vi "OSSCAR_v3_BM.vi"() -> ()   [LabVIEW 2021]
uses:
  SubVIs/Global_stop.vi
  SubVIs/Plot_trap_heating_global_BM.vi
  SubVIs/OSSCAR_stop_global_BM.vi
  SubVIs/DMSO-related/Temp_global_BM.vi
panel:
  in  "N Interval Pt. Std.s":dbl=6.0 caption="Every"
  in  "Interval Pt. Std.?":bool
  in  "Runtype":enum16{"Single", "Continuous"}(ring)
  in  "Program Control":bool caption="Program Stop"
  out "Current Std #":string
  out "Current Analyte:":string="DMS"
  in  "N std pt.s":i32=6
  in  "Mode Selection":T1(ring)
  in  "Standalone Function":T2(ring)=enum."Condition Trap"
  out "Reduction Countdown (min)":dbl format="%.2g"
  out "Hydrolysis Countdown (min)":dbl format="%.2g"
  out "Sparge Countdown (min)":dbl format="%.2g"
  out "Elution Countdown (min)":dbl format="%.2f"
  out "Hydrolysis Progress Bar":u8(slide)=100 scale=0.0..100.0
  out "Reduction Progress Bar":u8(slide)=100 scale=0.0..100.0
  out "Elution Progress Bar":u8(slide)=100 scale=0.0..100.0
  out "Sparging Progress Bar":u8(slide)=100 scale=0.0..100.0
  in  "Analysis Type":T3(ring)
  in  "Tab Control":T4(tab)
  in  "Metadata":T5={"Local save location:"="C:\\Users\\LabPC1\\OneDrive\\Desktop\\OSSCAR_metadata\\Test_metadata", "Cruise ID"="LaPerouse", "Sampling Timestamp"="2023-07-19 15:23:13", "Elution Timestamp"="2023-07-19 15:29:12", "GPS_Latitude"=-999.0, "GPS_Longitude"=-999.0, "DMS_std_conc"=0.0, "DMSP_std_conc"=0.0, "DMSO_std_conc"=0.0, "Std_index"=0.0, "Initial Trap Temp (oC)"=29.0, "Max Trap Temp (oC)"=161.0, "Final Trap Temp (oC)"=31.0, "Flow Rate (mL/min)"=0.0, "Comment"="", "GPS_Minute"=-999.0, "GPS_Day"=-999.0, "GPS_jd"=-999.0, "GPS_Hour"=-999.0, "GPS_Second"=-999.0, "GPS Baud"=4800.0, "COM Port (GPS)"="COM10", "Use GPS?"=FALSE, "Format Date"="%d-%d-%d"} {"GPS_Latitude" format="%_4g"; "GPS_Longitude" format="%_4g"; "GPS_jd" format="%_5g"; "Std_index" format="%.2g"; "DMSO_std_conc" format="%.2f"; "DMSP_std_conc" format="%.2f"; "DMS_std_conc" format="%.2f"}
  in  "Sample Params":T6={"DMS Sparge Time (min)"=7.0, "Elution Time (min)"=1.5, "COM port (16 Pos. Valve)"="COM10", "Trap Heating Time (ms)"=900.0, "COM Port (DC Power)"="COM5", "COM Port (Runze)"="COM4", "Sample Vol (mL)"=10.0, "DMSO Red. Duration (min)"=30.0, "Bypass sample handling (debugging)"=FALSE, "Reverse Reduction?"=FALSE, "Voltage (V)"="4.0", "DMSP Hydrolysis Time (min)"=13.0, "Total Vol. (mL)"=10.0, "Split DMSP sample?"=TRUE, "Remove DMSP vol. (mL)"=5.0}
  in  "Constants":T7={"step to ml"=1920.0, "BoardNum"=0, "PosA BitNum"=1, "PosB BitNum"=2, "Heat Pulse Delay (ms)"=0.0, "Heating Iterations"=12, "N rinses"=2, "Dissolution Time (s)"=120, "SpargeBit"=0, "Extra Milli-Q (ml)"=2.0, "Valco Port Number"=6, "BitNum (Thermocouple)"=1, "N syringe rinses"=2, "NaOH Vol (ml)"=2.0, "FanBit"=4}
  in  "Pump Parameters":T8={"Speed 1"="100", "Speed 2"="250", "Speed 3"="350", "Speed 4"="250", "UW/Sample"="5", "Sparge"="2", "Std"="4", "Waste"="15", "Air"="14", "Milli-Q"="1", "H2SO4"="6", "NaOH"="3", "Catalyst"="7", "Cell (H+ side)"="8", "Cell (sample side)"="9", "NaCl"="11"}
  out "Current Temp:":i32=31
  out "Trap Heating":cluster{"Y":dbl[], "Y":dbl[]}[](graph)
  # "OSSCAR DMS/O/P Program"
  # "Runs"
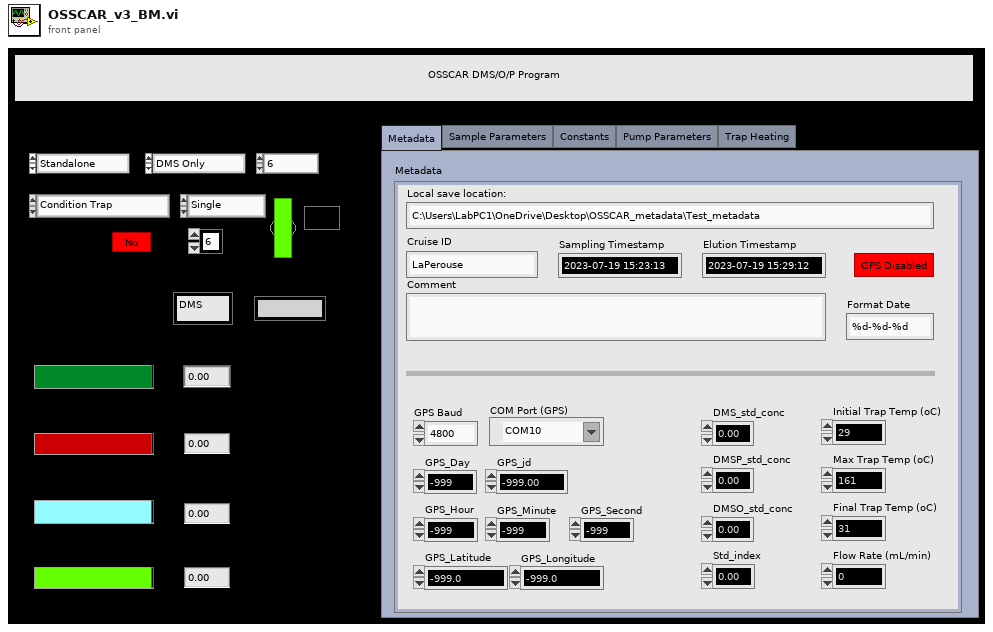
[diagram p1: front panel]
types:
  T1 = enum16{"Standalone", "Analysis", "Standard Curve", "Point Std"}
  T2 = enum16{"Send Pump Command", "Condition Trap", "Control Fan", "Control Sparger", "Load/Inject Trap", "Switch Flow Path", "Control cell DC power", "Rinse Sparge Chamber", "Rinse Cell"}
  T3 = enum16{"DMS Only", "DMS/O", "DMS/P", "DMS/O/P", "DMSO Only"}
  T4 = enum32{"Metadata", "Sample Parameters", "Constants", "Pump Parameters", "Trap Heating"}
  T5 = cluster{"Local save location:":string, "Cruise ID":string, "Sampling Timestamp":string, "Elution Timestamp":string, "GPS_Latitude":dbl, "GPS_Longitude":dbl, "DMS_std_conc":dbl, "DMSP_std_conc":dbl, "DMSO_std_conc":dbl, "Std_index":dbl, "Initial Trap Temp (oC)":dbl, "Max Trap Temp (oC)":dbl, "Final Trap Temp (oC)":dbl, "Flow Rate (mL/min)":dbl, "Comment":string, "GPS_Minute":dbl, "GPS_Day":dbl, "GPS_jd":dbl, "GPS_Hour":dbl, "GPS_Second":dbl, "GPS Baud":dbl, "COM Port (GPS)":refnum<visa-resource-name>, "Use GPS?":bool, "Format Date":string}
  T6 = cluster{"DMS Sparge Time (min)":dbl, "Elution Time (min)":dbl, "COM port (16 Pos. Valve)":refnum<visa-resource-name>, "Trap Heating Time (ms)":dbl, "COM Port (DC Power)":refnum<visa-resource-name>, "COM Port (Runze)":refnum<visa-resource-name>, "Sample Vol (mL)":dbl, "DMSO Red. Duration (min)":dbl, "Bypass sample handling (debugging)":bool, "Reverse Reduction?":bool, "Voltage (V)":string, "DMSP Hydrolysis Time (min)":dbl, "Total Vol. (mL)":dbl, "Split DMSP sample?":bool, "Remove DMSP vol. (mL)":dbl}
  T7 = cluster{"step to ml":dbl, "BoardNum":u32, "PosA BitNum":u32, "PosB BitNum":u32, "Heat Pulse Delay (ms)":dbl, "Heating Iterations":i32, "N rinses":i32, "Dissolution Time (s)":u32, "SpargeBit":u32, "Extra Milli-Q (ml)":dbl, "Valco Port Number":i32, "BitNum (Thermocouple)":u32, "N syringe rinses":i32, "NaOH Vol (ml)":dbl, "FanBit":u32}
  T8 = cluster{"Speed 1":string, "Speed 2":string, "Speed 3":string, "Speed 4":string, "UW/Sample":string, "Sparge":string, "Std":string, "Waste":string, "Air":string, "Milli-Q":string, "H2SO4":string, "NaOH":string, "Catalyst":string, "Cell (H+ side)":string, "Cell (sample side)":string, "NaCl":string}
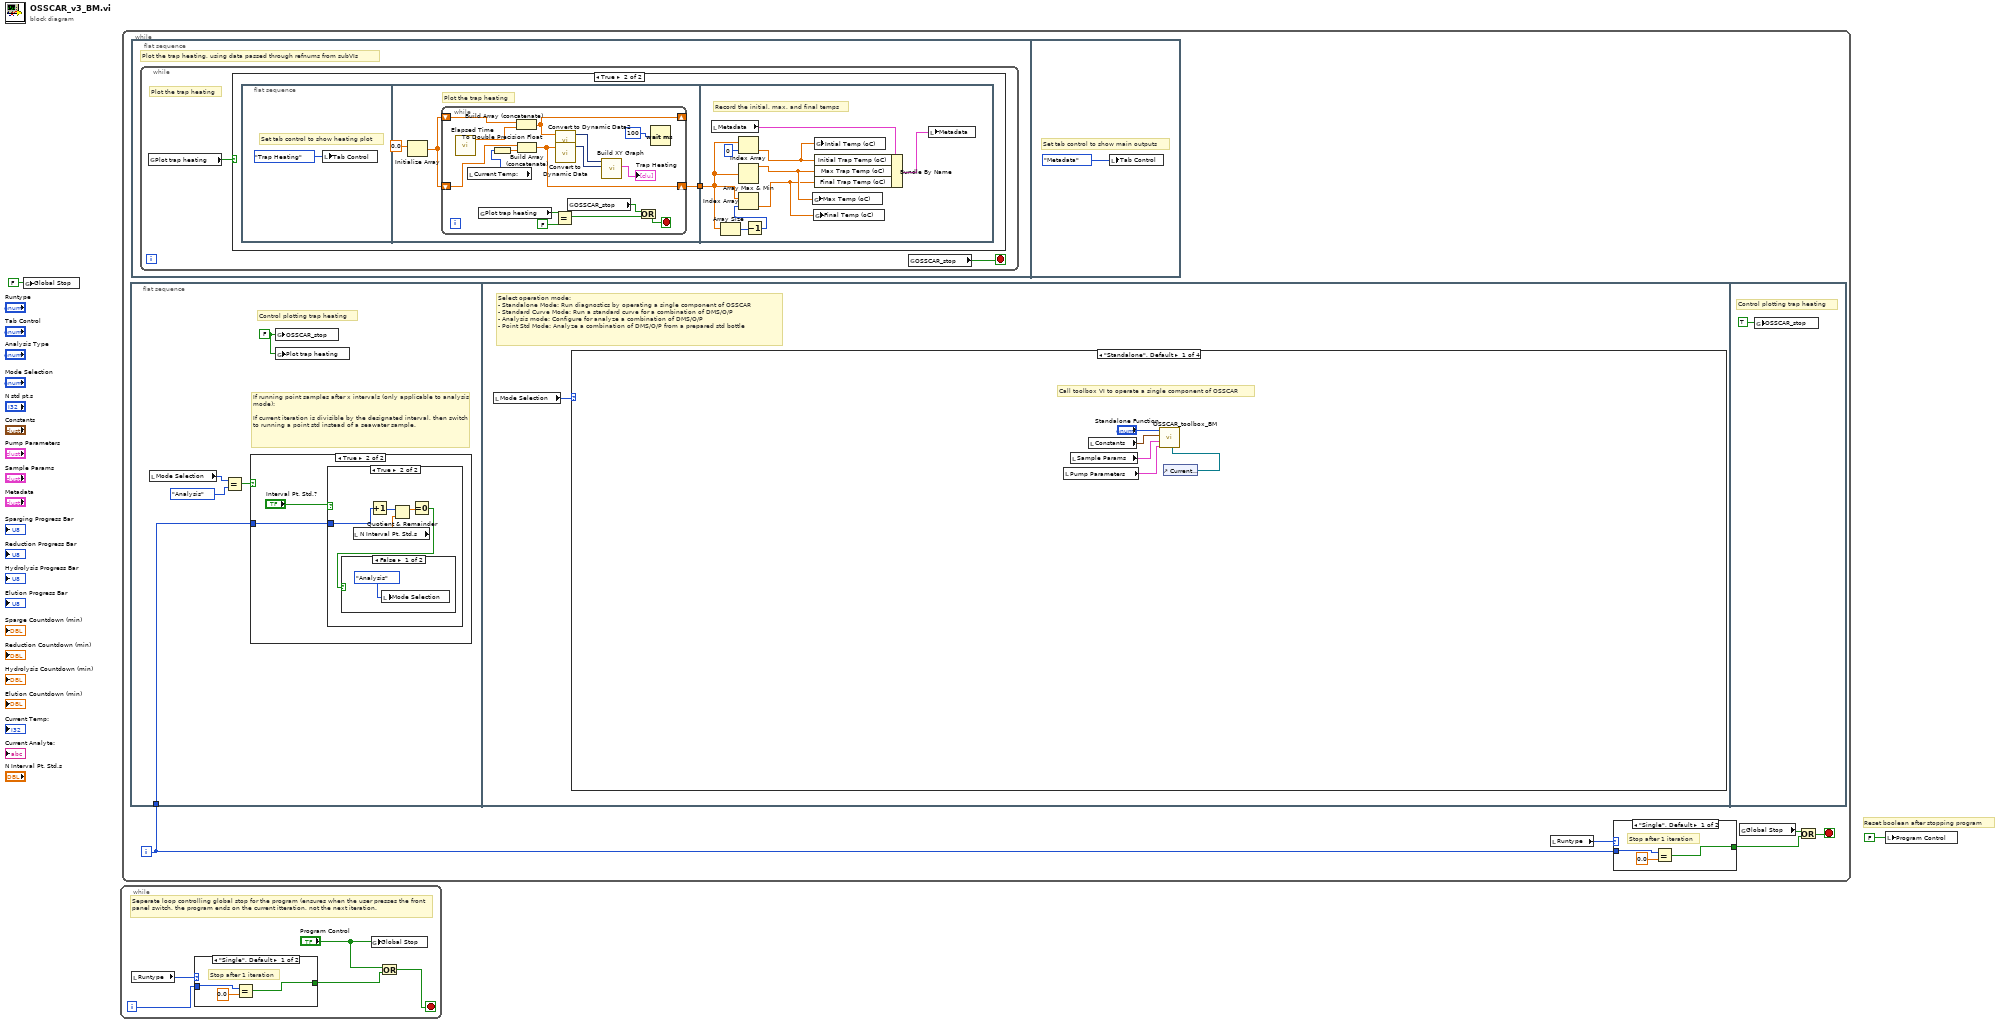
[diagram p0: block diagram]
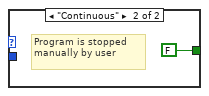
[diagram p2: hidden frame]
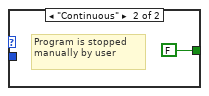
[diagram p4: hidden frame]
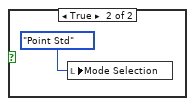
[diagram p7: hidden frame]
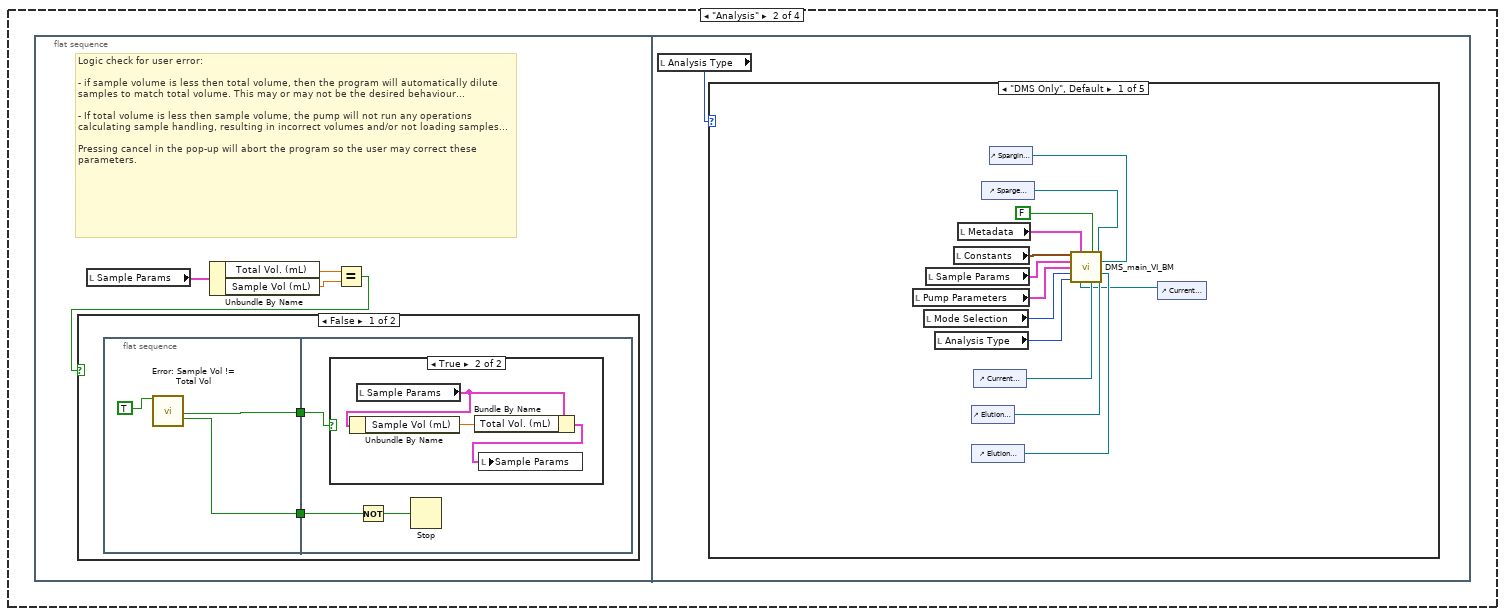
[diagram p8: hidden frame]
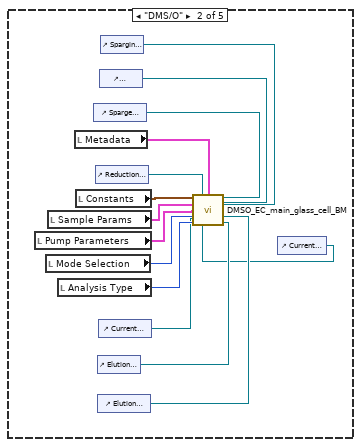
[diagram p11: hidden frame]
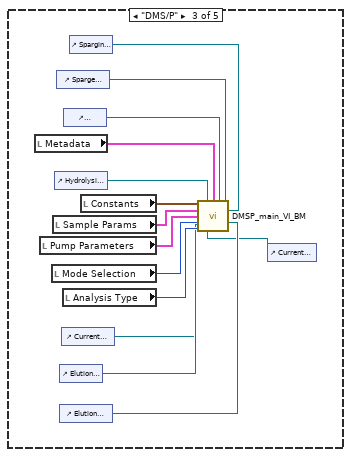
[diagram p12: hidden frame]
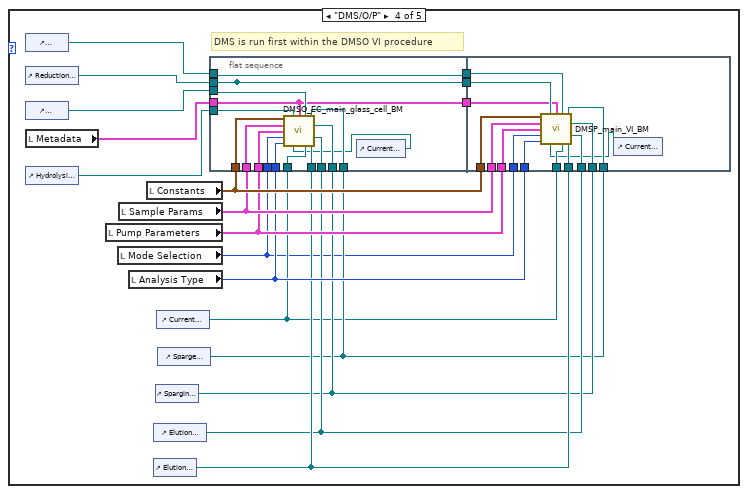
[diagram p13: hidden frame]
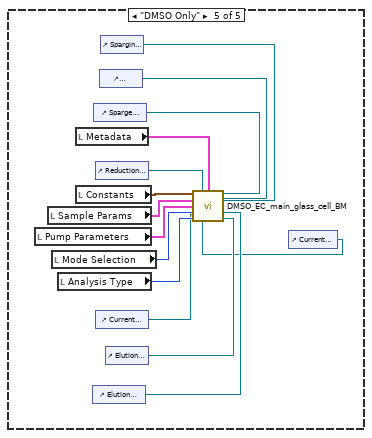
[diagram p14: hidden frame]
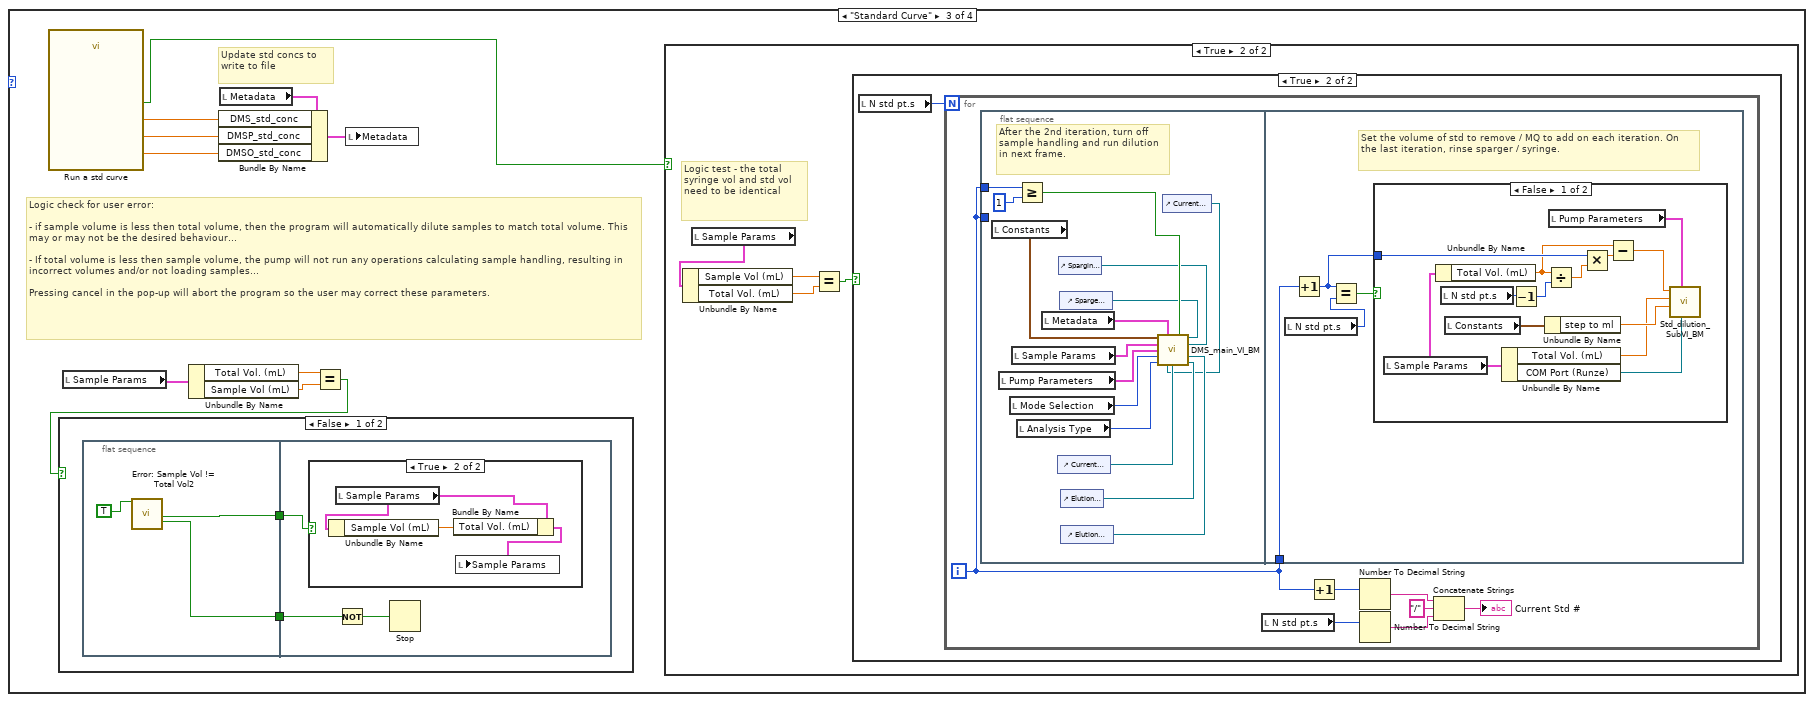
[diagram p15: hidden frame]
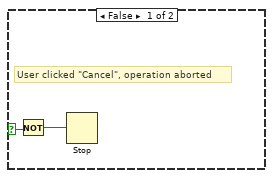
[diagram p18: hidden frame]
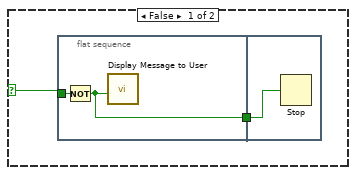
[diagram p19: hidden frame]
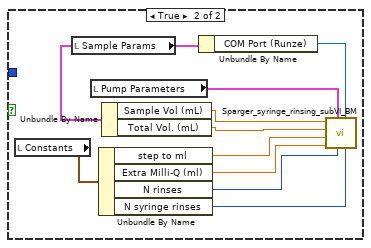
[diagram p20: hidden frame]
diagram:
  # "Reset boolean after stopping program"
  n1 = global write "Global_stop.vi" "Global Stop"(FALSE ("Global Stop")) -> ()
  n2 = while {
    i -> [w3]
    stop <- w4 stop-if-true
    # "Seperate loop controlling global stop for the program (ensures when the user presses the front panel switch, the program ends on the current itteration, not the next iteration."
    n3 = local read "Runtype"() -> (w7:enum16{"Single", "Continuous"})
    n4 = case shown="\"Single\", Default" w7 {
      tunnel: w3 -> [w9 _]
      tunnel: [w8 FALSE] -> w6
      frame "Single", Default {
        # "Stop after 1 iteration"
        n5 = Equal?(x=w9, y=0.0) -> (x = y?=w8:bool)
      }
      frame "Continuous" {
        # "Program is stopped manually by user"
      }
    }
    n6 = global write "Global_stop.vi" "Global Stop"("Program Control") -> ()
    n7 = Or(x="Program Control", y=w6) -> (x .or. y?=w4:bool)
  }
  n8 = while {
    i -> [w15]
    stop <- w14 stop-if-true
    n9 = flat-sequence {
      tunnel: w15 -> [w57]
      frame #0 {
        w58 = FALSE ("OSSCAR_stop")
        # "If running point samples after x intervals (only applicable to analysis mode):\n\nIf current iteration is divisible by the designated interval, then switch to running a point std instead of a seawater sample."
        # "Control plotting trap heating"
        n10 = local read "Mode Selection"() -> (w55:T1)
        n11 = Equal?(x=w55, y=T1."Analysis" ("Mode Selection")) -> (x = y?=w56:bool)
        n12 = case shown="True" w56 {
          tunnel: w57 -> [_ w60]
          frame False {
            # "Not running analysis / point std, proceed with other operations"
          }
          frame True {
            n13 = case shown="True" "Interval Pt. Std.?" {
              tunnel: w60 -> [_ w61]
              frame False {
                # "Not running point stds, so continue with analysis"
              }
              frame True {
                n14 = local read "N Interval Pt. Std.s"() -> (w65:dbl)
                n15 = Increment(x=w61) -> (x+1=w62:i32)
                n16 = Quotient & Remainder(x=w62, y=w65) -> (x-y*floor(x/y)=w64:dbl)  [unwired: 1 out]
                n17 = Equal To 0?(x=w64) -> (x = 0?=w63:bool)
                n18 = case shown="False" w63 {
                  frame False {
                    n19 = local write "Mode Selection"(T1."Analysis" ("Mode Selection")) -> ()
                  }
                  frame True {
                    n20 = local write "Mode Selection"(T1."Point Std" ("Mode Selection")) -> ()
                  }
                }
              }
            }
          }
        }
        n21 = global write "OSSCAR_stop_global_BM.vi" "OSSCAR_stop"(w58) -> ()
        n22 = global write "Plot_trap_heating_global_BM.vi" "Plot trap heating"(w58) -> ()
      }
      frame #1 {
        # "Select operation mode:\n- Standalone Mode: Run diagnostics by operating a single component of OSSCAR\n- Standard Curve Mode: Run a standard curve for a combination of DMS/O/P\n- Analysis mode: Configure for analyze a combination of DMS/O/P\n- Point Std Mode: Analyze a combination of DMS/O/P from a prepared std bottle"
        n23 = local read "Mode Selection"() -> (w68:T1)
        n24 = case shown="\"Standalone\", Default" w68 {
          frame "Standalone", Default {
            # "Call toolbox VI to operate a single component of OSSCAR"
            n25 = local read "Pump Parameters"() -> (w69:T8)
            n26 = local read "Sample Params"() -> (w70:T6)
            n27 = local read "Constants"() -> (w71:T7)
            n28 = control-ref of="Current Temp:"() -> (w72:refnum<vi>)
            n29 = call "OSSCAR_toolbox_BM.vi"("Temp Refnum"=w72, "Pump Parameters"=w69, "Sample Params"=w70, "Constants"=w71, "Function"="Standalone Function") -> ()  [unwired: 7 in]
          }
          frame "Analysis" {
            n30 = flat-sequence {
              frame #0 {
                # "Logic check for user error:\n\n- if sample volume is less then total volume, then the program will automatically dilute samples to match total volume. This may or may not be the desired behaviour...\n\n- If total volume is less then sample volume, the pump will not run any operations calculating sample handling, resulting in incorrect volumes and/or not loading samples...\n\nPressing cancel in the pop-up will abort the program so the user may correct these parameters."
                n31 = local read "Sample Params"() -> (w77:T6)
                n32 = Unbundle By Name(w77) -> ("Total Vol. (mL)"=w74:dbl, "Sample Vol (mL)"=w76:dbl)
                n33 = Equal?(x=w74, y=w76) -> (x = y?=w75:bool)
                n34 = case shown="False" w75 {
                  frame False {
                    n35 = flat-sequence {
                      tunnel: [w82] -> w79
                      tunnel: [w81] -> w78
                      tunnel: w79 -> [w85]
                      tunnel: w78 -> [w83]
                      frame #0 {
                        n36 = call "Error: Sample Vol != Total Vol"("Enable"=TRUE) -> ("Make Total Vol = Sample Vol?"=w81:bool, "Proceed"=w82:bool)  [unwired: 16 in, 1 out]
                      }
                      frame #1 {
                        n37 = case shown="True" w83 {
                          frame False {
                            # "User indicated sample vol should not equal total vol, continue to analysis."
                          }
                          frame True {
                            n38 = local read "Sample Params"() -> (w87:T6)
                            n39 = Unbundle By Name(w87) -> ("Sample Vol (mL)"=w88:dbl)
                            n40 = Bundle By Name(cluster=w87, "Total Vol. (mL)"=w88) -> (w86:T6)
                            n41 = local write "Sample Params"(w86) -> ()
                          }
                        }
                        n42 = Not(x=w85) -> (.not. x?=w84:bool)
                        n43 = Stop(stop? (T)=w84) -> ()
                      }
                    }
                  }
                  frame True {
                    # "Else: carry on, nothing to see here..."
                  }
                }
              }
              frame #1 {
                n44 = local read "Analysis Type"() -> (w89:T3)
                n45 = case shown="\"DMS Only\", Default" w89 {
                  frame "DMS Only", Default {
                    n46 = local read "Pump Parameters"() -> (w101:T8)
                    n47 = local read "Mode Selection"() -> (w90:T1)
                    n48 = local read "Sample Params"() -> (w102:T6)
                    n49 = local read "Analysis Type"() -> (w100:T3)
                    n50 = local read "Constants"() -> (w93:T7)
                    n51 = local read "Metadata"() -> (w92:T5)
                    n52 = control-ref of="Elution Progress Bar"() -> (w95:refnum<vi>)
                    n53 = control-ref of="Elution Countdown (min)"() -> (w96:refnum<vi>)
                    n54 = control-ref of="Current Temp:"() -> (w94:refnum<vi>)
                    n55 = control-ref of="Sparge Countdown (min)"() -> (w98:refnum<vi>)
                    n56 = control-ref of="Sparging Progress Bar"() -> (w97:refnum<vi>)
                    n57 = control-ref of="Current Analyte:"() -> (w91:refnum<vi>)
                    n58 = call "DMS_main_VI_BM.vi"("Constants"=w93, "Metadata"=w92, "Skip sample handling"=FALSE, "Sparging Countdown Timer Refnum"=w98, "Sample Params"=w102, "Sparging Progress Bar Refnum"=w97, "Pump Parameters"=w101, "Mode Selection"=w90, "Elution Countdown Timer Refnum"=w96, "Analysis Type"=w100, "Current Analyte Refnum"=w91, "Temp Refnum"=w94, "Elution Progress Bar Refnum"=w95) -> ()  [unwired: 3 in]
                  }
                  frame "DMS/O" {
                    n59 = local read "Pump Parameters"() -> (w104:T8)
                    n60 = local read "Mode Selection"() -> (w103:T1)
                    n61 = local read "Sample Params"() -> (w115:T6)
                    n62 = local read "Analysis Type"() -> (w116:T3)
                    n63 = local read "Metadata"() -> (w106:T5)
                    n64 = local read "Constants"() -> (w107:T7)
                    n65 = control-ref of="Sparge Countdown (min)"() -> (w112:refnum<vi>)
                    n66 = control-ref of="Reduction Countdown (min)"() -> (w114:refnum<vi>)
                    n67 = control-ref of="Elution Progress Bar"() -> (w110:refnum<vi>)
                    n68 = control-ref of="Elution Countdown (min)"() -> (w109:refnum<vi>)
                    n69 = control-ref of="Current Temp:"() -> (w108:refnum<vi>)
                    n70 = control-ref of="Reduction Progress Bar"() -> (w113:refnum<vi>)
                    n71 = control-ref of="Sparging Progress Bar"() -> (w111:refnum<vi>)
                    n72 = control-ref of="Current Analyte:"() -> (w105:refnum<vi>)
                    n73 = call "DMSO_EC_main_glass_cell_BM.vi"("Constants"=w107, "Reduction Countdown Timer Refnum"=w114, "Metadata"=w106, "Reduction Progress Bar Refnum"=w113, "Sparging Countdown Timer Refnum"=w112, "Sample Params"=w115, "Sparging Progress Bar Refnum"=w111, "Pump Parameters"=w104, "Mode Selection"=w103, "Elution Countdown Timer Refnum"=w109, "Analysis Type"=w116, "Current Analyte Refnum"=w105, "Temp Refnum"=w108, "Elution Progress Bar Refnum"=w110) -> ()  [unwired: 2 in]
                  }
                  frame "DMS/P" {
                    n74 = local read "Metadata"() -> (w120:T5)
                    n75 = local read "Pump Parameters"() -> (w118:T8)
                    n76 = local read "Mode Selection"() -> (w117:T1)
                    n77 = local read "Sample Params"() -> (w129:T6)
                    n78 = control-ref of="Hydrolysis Countdown (min)"() -> (w125:refnum<vi>)
                    n79 = control-ref of="Sparge Countdown (min)"() -> (w123:refnum<vi>)
                    n80 = control-ref of="Elution Progress Bar"() -> (w127:refnum<vi>)
                    n81 = control-ref of="Elution Countdown (min)"() -> (w128:refnum<vi>)
                    n82 = control-ref of="Current Temp:"() -> (w122:refnum<vi>)
                    n83 = local read "Analysis Type"() -> (w130:T3)
                    n84 = control-ref of="Hydrolysis Progress Bar"() -> (w126:refnum<vi>)
                    n85 = control-ref of="Sparging Progress Bar"() -> (w124:refnum<vi>)
                    n86 = local read "Constants"() -> (w121:T7)
                    n87 = control-ref of="Current Analyte:"() -> (w119:refnum<vi>)
                    n88 = call "DMSP_main_VI_BM.vi"("Constants"=w121, "Hydrolysis Countdown Refnum"=w125, "Metadata"=w120, "Hydrolysis Progress Bar Refnum"=w126, "Sparge Countdown Timer Refnum"=w123, "Sample Params"=w129, "Sparging Progress Bar Refnum"=w124, "Pump Parameters"=w118, "Mode Selection"=w117, "Elution Countdown Timer Refnum"=w128, "Analysis Type"=w130, "Current Analyte Refnum"=w119, "Temp Refnum"=w122, "Elution Progress Bar Refnum"=w127) -> ()  [unwired: 2 in]
                  }
                  frame "DMS/O/P" {
                    # "DMS is run first within the DMSO VI procedure"
                    n89 = control-ref of="Reduction Progress Bar"() -> (w139:refnum<vi>)
                    n90 = control-ref of="Reduction Countdown (min)"() -> (w141:refnum<vi>)
                    n91 = control-ref of="Hydrolysis Progress Bar"() -> (w143:refnum<vi>)
                    n92 = local read "Metadata"() -> (w133:T5)
                    n93 = control-ref of="Hydrolysis Countdown (min)"() -> (w144:refnum<vi>)
                    n94 = local read "Pump Parameters"() -> (w146:T8)
                    n95 = local read "Mode Selection"() -> (w131:T1)
                    n96 = local read "Sample Params"() -> (w147:T6)
                    n97 = local read "Analysis Type"() -> (w145:T3)
                    n98 = local read "Constants"() -> (w148:T7)
                    n99 = control-ref of="Elution Countdown (min)"() -> (w137:refnum<vi>)
                    n100 = control-ref of="Elution Progress Bar"() -> (w138:refnum<vi>)
                    n101 = control-ref of="Sparging Progress Bar"() -> (w136:refnum<vi>)
                    n102 = control-ref of="Current Temp:"() -> (w134:refnum<vi>)
                    n103 = control-ref of="Sparge Countdown (min)"() -> (w135:refnum<vi>)
                    n104 = flat-sequence {
                      tunnel: w148 -> [w153]
                      tunnel: w147 -> [w164]
                      tunnel: w146 -> [w150]
                      tunnel: w145 -> [w163]
                      tunnel: w144 -> [w162]
                      tunnel: w143 -> [w161]
                      tunnel: [w160] -> _
                      tunnel: [w160] -> w142
                      tunnel: w141 -> [w160]
                      tunnel: w139 -> [w159]
                      tunnel: [w159] -> w140
                      tunnel: w135 -> [w158]
                      tunnel: w136 -> [w157]
                      tunnel: w137 -> [w156]
                      tunnel: w138 -> [w155]
                      tunnel: w134 -> [w154]
                      tunnel: w133 -> [w152]
                      tunnel: [w152] -> w132
                      tunnel: w131 -> [w149]
                      tunnel: w148 -> [w169]
                      tunnel: w147 -> [w178]
                      tunnel: w146 -> [w166]
                      tunnel: w145 -> [w177]
                      tunnel: w142 -> [w176]
                      tunnel: w140 -> [w175]
                      tunnel: w138 -> [w174]
                      tunnel: w137 -> [w173]
                      tunnel: w136 -> [w172]
                      tunnel: w135 -> [w171]
                      tunnel: w134 -> [w170]
                      tunnel: w132 -> [w168]
                      tunnel: w131 -> [w165]
                      frame #0 {
                        n105 = control-ref of="Current Analyte:"() -> (w151:refnum<vi>)
                        n106 = call "DMSO_EC_main_glass_cell_BM.vi"("Constants"=w153, "Reduction Countdown Timer Refnum"=w162, "Metadata"=w152, "Reduction Progress Bar Refnum"=w161, "Sparging Countdown Timer Refnum"=w158, "Sample Params"=w164, "Sparging Progress Bar Refnum"=w157, "Pump Parameters"=w150, "Mode Selection"=w149, "Elution Countdown Timer Refnum"=w156, "Analysis Type"=w163, "Current Analyte Refnum"=w151, "Temp Refnum"=w154, "Elution Progress Bar Refnum"=w155) -> ()  [unwired: 2 in]
                      }
                      frame #1 {
                        n107 = control-ref of="Current Analyte:"() -> (w167:refnum<vi>)
                        n108 = call "DMSP_main_VI_BM.vi"("Constants"=w169, "Hydrolysis Countdown Refnum"=w176, "Metadata"=w168, "Hydrolysis Progress Bar Refnum"=w175, "Sparge Countdown Timer Refnum"=w171, "Sample Params"=w178, "Sparging Progress Bar Refnum"=w172, "Pump Parameters"=w166, "Mode Selection"=w165, "Elution Countdown Timer Refnum"=w173, "Analysis Type"=w177, "Current Analyte Refnum"=w167, "Temp Refnum"=w170, "Elution Progress Bar Refnum"=w174) -> ()  [unwired: 2 in]
                      }
                    }
                  }
                  frame "DMSO Only" {
                    n109 = local read "Pump Parameters"() -> (w180:T8)
                    n110 = local read "Sample Params"() -> (w191:T6)
                    n111 = local read "Mode Selection"() -> (w179:T1)
                    n112 = local read "Analysis Type"() -> (w192:T3)
                    n113 = local read "Metadata"() -> (w182:T5)
                    n114 = local read "Constants"() -> (w183:T7)
                    n115 = control-ref of="Elution Countdown (min)"() -> (w185:refnum<vi>)
                    n116 = control-ref of="Sparge Countdown (min)"() -> (w188:refnum<vi>)
                    n117 = control-ref of="Reduction Countdown (min)"() -> (w190:refnum<vi>)
                    n118 = control-ref of="Current Temp:"() -> (w184:refnum<vi>)
                    n119 = control-ref of="Reduction Progress Bar"() -> (w189:refnum<vi>)
                    n120 = control-ref of="Sparging Progress Bar"() -> (w187:refnum<vi>)
                    n121 = control-ref of="Elution Progress Bar"() -> (w186:refnum<vi>)
                    n122 = control-ref of="Current Analyte:"() -> (w181:refnum<vi>)
                    n123 = call "DMSO_EC_main_glass_cell_BM.vi"("Constants"=w183, "Reduction Countdown Timer Refnum"=w190, "Metadata"=w182, "Reduction Progress Bar Refnum"=w189, "Sparging Countdown Timer Refnum"=w188, "Sample Params"=w191, "Sparging Progress Bar Refnum"=w187, "Pump Parameters"=w180, "Mode Selection"=w179, "Elution Countdown Timer Refnum"=w185, "Analysis Type"=w192, "Current Analyte Refnum"=w181, "Temp Refnum"=w184, "Elution Progress Bar Refnum"=w186) -> ()  [unwired: 2 in]
                  }
                }
              }
            }
          }
          frame "Standard Curve" {
            # "Logic check for user error:\n\n- if sample volume is less then total volume, then the program will automatically dilute samples to match total volume. This may or may not be the desired behaviour...\n\n- If total volume is less then sample volume, the pump will not run any operations calculating sample handling, resulting in incorrect volumes and/or not loading samples...\n\nPressing cancel in the pop-up will abort the program so the user may correct these parameters."
            # "Update std concs to write to file"
            n124 = call "Run a std curve"() -> ("DMSO std concentration"=w199:dbl, "DMSP std concentration"=w198:dbl, "DMS std concentration"=w197:dbl, "OK"=w202:bool)  [unwired: 15 in, 1 out]
            n125 = local read "Sample Params"() -> (w196:T6)
            n126 = Unbundle By Name(w196) -> ("Total Vol. (mL)"=w193:dbl, "Sample Vol (mL)"=w195:dbl)
            n127 = local read "Metadata"() -> (w201:T5)
            n128 = Bundle By Name(cluster=w201, "DMS_std_conc"=w197, "DMSP_std_conc"=w198, "DMSO_std_conc"=w199) -> (w200:T5)
            n129 = Equal?(x=w193, y=w195) -> (x = y?=w194:bool)
            n130 = case shown="False" w194 {
              frame False {
                n131 = flat-sequence {
                  tunnel: [w207] -> w204
                  tunnel: [w206] -> w203
                  tunnel: w204 -> [w210]
                  tunnel: w203 -> [w208]
                  frame #0 {
                    n132 = call "Error: Sample Vol != Total Vol2"("Enable"=TRUE) -> ("Make Total Vol = Sample Vol?"=w206:bool, "Proceed"=w207:bool)  [unwired: 16 in, 1 out]
                  }
                  frame #1 {
                    n133 = case shown="True" w208 {
                      frame False {
                        # "User indicated sample vol should not equal total vol, continue to analysis."
                      }
                      frame True {
                        n134 = local read "Sample Params"() -> (w213:T6)
                        n135 = Unbundle By Name(w213) -> ("Sample Vol (mL)"=w212:dbl)
                        n136 = Bundle By Name(cluster=w213, "Total Vol. (mL)"=w212) -> (w211:T6)
                        n137 = local write "Sample Params"(w211) -> ()
                      }
                    }
                    n138 = Not(x=w210) -> (.not. x?=w209:bool)
                    n139 = Stop(stop? (T)=w209) -> ()
                  }
                }
              }
              frame True {
                # "Else: carry on, nothing to see here..."
              }
            }
            n140 = local write "Metadata"(w200) -> ()
            n141 = case shown="True" w202 {
              selector: w202 -> [w214 _]
              frame False {
                # "User clicked \"Cancel\", operation aborted"
                n142 = Not(x=w214) -> (.not. x?=w215:bool)
                n143 = Stop(stop? (T)=w215) -> ()
              }
              frame True {
                # "Logic test - the total syringe vol and std vol need to be identical"
                n144 = local read "Sample Params"() -> (w219:T6)
                n145 = Unbundle By Name(w219) -> ("Sample Vol (mL)"=w217:dbl, "Total Vol. (mL)"=w216:dbl)
                n146 = Equal?(x=w217, y=w216) -> (x = y?=w218:bool)
                n147 = case shown="True" w218 {
                  selector: w218 -> [w220 _]
                  frame False {
                    n148 = flat-sequence {
                      tunnel: w220 -> [w223]
                      tunnel: [w222] -> w221
                      tunnel: w221 -> [w224]
                      frame #0 {
                        n149 = Not(x=w223) -> (.not. x?=w222:bool)
                        n150 = call "Display Message to User"("Enable"=w222) -> ()  [unwired: 9 in, 2 out]
                      }
                      frame #1 {
                        n151 = Stop(stop? (T)=w224) -> ()
                      }
                    }
                  }
                  frame True {
                    n152 = local read "N std pt.s"() -> (w225:i32)
                    n153 = for {
                      N: w225 -> [_]
                      i -> [w232]
                      n154 = flat-sequence {
                        tunnel: w232 -> [w247]
                        tunnel: w232 -> [_]
                        tunnel: w232 -> [w250]
                        frame #0 {
                          # "After the 2nd iteration, turn off sample handling and run dilution in next frame."
                          n155 = local read "Constants"() -> (w236:T7)
                          n156 = local read "Pump Parameters"() -> (w244:T8)
                          n157 = local read "Mode Selection"() -> (w233:T1)
                          n158 = local read "Sample Params"() -> (w243:T6)
                          n159 = Greater Or Equal?(x=w247, y=1) -> (x >= y?=w242:bool)
                          n160 = local read "Analysis Type"() -> (w245:T3)
                          n161 = local read "Metadata"() -> (w235:T5)
                          n162 = control-ref of="Current Temp:"() -> (w237:refnum<vi>)
                          n163 = control-ref of="Sparging Progress Bar"() -> (w240:refnum<vi>)
                          n164 = control-ref of="Sparge Countdown (min)"() -> (w241:refnum<vi>)
                          n165 = control-ref of="Elution Progress Bar"() -> (w238:refnum<vi>)
                          n166 = control-ref of="Elution Countdown (min)"() -> (w239:refnum<vi>)
                          n167 = control-ref of="Current Analyte:"() -> (w234:refnum<vi>)
                          n168 = call "DMS_main_VI_BM.vi"("Constants"=w236, "Metadata"=w235, "Skip sample handling"=w242, "Sparging Countdown Timer Refnum"=w241, "Sample Params"=w243, "Sparging Progress Bar Refnum"=w240, "Pump Parameters"=w244, "Mode Selection"=w233, "Elution Countdown Timer Refnum"=w239, "Analysis Type"=w245, "Current Analyte Refnum"=w234, "Temp Refnum"=w237, "Elution Progress Bar Refnum"=w238) -> ()  [unwired: 3 in]
                        }
                        frame #1 {
                          # "Set the volume of std to remove / MQ to add on each iteration. On the last iteration, rinse sparger / syringe."
                          n169 = local read "N std pt.s"() -> (w249:i32)
                          n170 = Increment(x=w250) -> (x+1=w248:i32)
                          n171 = Equal?(x=w248, y=w249) -> (x = y?=w251:bool)
                          n172 = case shown="False" w251 {
                            tunnel: w248 -> [w260 _]
                            frame False {
                              n173 = local read "Sample Params"() -> (w254:T6)
                              n174 = Unbundle By Name(w254) -> ("Total Vol. (mL)"=w253:dbl)
                              n175 = local read "N std pt.s"() -> (w261:i32)
                              n176 = local read "Constants"() -> (w258:T7)
                              n177 = Unbundle By Name(w254) -> ("Total Vol. (mL)"=w252:dbl, "COM Port (Runze)"=w256:refnum<visa-resource-name>)
                              n178 = Decrement(x=w261) -> (x-1=w262:i32)
                              n179 = Unbundle By Name(w258) -> ("step to ml"=w257:dbl)
                              n180 = Divide(x=w253, y=w262) -> (x/y=w263:dbl)
                              n181 = local read "Pump Parameters"() -> (w255:T8)
                              n182 = Multiply(x=w260, y=w263) -> (x*y=w264:dbl)
                              n183 = Subtract(x=w253, y=w264) -> (x-y=w259:dbl)
                              n184 = call "Std_dilution_SubVI_BM.vi"("COM Port"=w256, "Pump Parameters"=w255, "step to ml"=w257, "Total Vol. (mL)"=w252, "Dilution Vol. (mL)"=w259) -> ()  [unwired: 7 in]
                            }
                            frame True {
                              n185 = local read "Constants"() -> (w266:T7)
                              n186 = local read "Sample Params"() -> (w267:T6)
                              n187 = local read "Pump Parameters"() -> (w269:T8)
                              n188 = Unbundle By Name(w266) -> ("step to ml"=w271:dbl, "Extra Milli-Q (ml)"=w272:dbl, "N rinses"=w273:i32, "N syringe rinses"=w274:i32)
                              n189 = Unbundle By Name(w267) -> ("Sample Vol (mL)"=w270:dbl, "Total Vol. (mL)"=w265:dbl)
                              n190 = Unbundle By Name(w267) -> ("COM Port (Runze)"=w268:refnum<visa-resource-name>)
                              n191 = call "Sparger_syringe_rinsing_subVI_BM.vi"("N syringe rinses"=w274, "COM Port"=w268, "N sparge rinses"=w273, "Pump Parameters"=w269, "Extra Milli-Q (ml)"=w272, "step to ml"=w271, "Total Vol. (mL)"=w265, "Sample Volume"=w270) -> ()  [unwired: 4 in]
                            }
                          }
                        }
                      }
                      n192 = local read "N std pt.s"() -> (w230:i32)
                      n193 = Increment(x=w232) -> (x+1=w231:i32)
                      n194 = Number To Decimal String(number=w231) -> (decimal integer string=w228:string)  [unwired: 1 in]
                      n195 = Number To Decimal String(number=w230) -> (decimal integer string=w227:string)  [unwired: 1 in]
                      n196 = Concatenate Strings(w228, "/" ("string"), w227) -> (→"Current Std #":string)
                    }
                  }
                }
              }
            }
          }
          frame "Point Std" {
            # "\"Point std\" operates the same as the normal analysis mode - only here, we draw sample from the \"std\" line instead of the seawater intake.  Note this mode allows individual (or mixed) DMS(/O/P) stds to be run, depending on the user's choice of \"Analysis Type\"."
            n197 = flat-sequence {
              frame #0 {
                # "Logic check for user error:\n\n- if sample volume is less then total volume, then the program will automatically dilute samples to match total volume. This may or may not be the desired behaviour...\n\n- If total volume is less then sample volume, the pump will not run any operations calculating sample handling, resulting in incorrect volumes and/or not loading samples...\n\nPressing cancel in the pop-up will abort the program so the user may correct these parameters."
                n198 = local read "Sample Params"() -> (w278:T6)
                n199 = Unbundle By Name(w278) -> ("Total Vol. (mL)"=w275:dbl, "Sample Vol (mL)"=w277:dbl)
                n200 = Equal?(x=w275, y=w277) -> (x = y?=w276:bool)
                n201 = case shown="False" w276 {
                  frame False {
                    n202 = flat-sequence {
                      tunnel: [w283] -> w280
                      tunnel: [w282] -> w279
                      tunnel: w280 -> [w286]
                      tunnel: w279 -> [w284]
                      frame #0 {
                        n203 = call "Error: Sample Vol != Total Vol3"("Enable"=TRUE) -> ("Make Total Vol = Sample Vol?"=w282:bool, "Proceed"=w283:bool)  [unwired: 16 in, 1 out]
                      }
                      frame #1 {
                        n204 = case shown="True" w284 {
                          frame False {
                            # "User indicated sample vol should not equal total vol, continue to analysis."
                          }
                          frame True {
                            n205 = local read "Sample Params"() -> (w288:T6)
                            n206 = Unbundle By Name(w288) -> ("Sample Vol (mL)"=w289:dbl)
                            n207 = Bundle By Name(cluster=w288, "Total Vol. (mL)"=w289) -> (w287:T6)
                            n208 = local write "Sample Params"(w287) -> ()
                          }
                        }
                        n209 = Not(x=w286) -> (.not. x?=w285:bool)
                        n210 = Stop(stop? (T)=w285) -> ()
                      }
                    }
                  }
                  frame True {
                    # "Else: carry on, nothing to see here..."
                  }
                }
              }
              frame #1 {
                n211 = local read "Analysis Type"() -> (w290:T3)
                n212 = case shown="\"DMS/O/P\"" w290 {
                  frame "DMS Only", Default {
                    n213 = local read "Pump Parameters"() -> (w302:T8)
                    n214 = local read "Mode Selection"() -> (w291:T1)
                    n215 = local read "Sample Params"() -> (w303:T6)
                    n216 = local read "Analysis Type"() -> (w301:T3)
                    n217 = local read "Constants"() -> (w294:T7)
                    n218 = local read "Metadata"() -> (w293:T5)
                    n219 = control-ref of="Elution Progress Bar"() -> (w296:refnum<vi>)
                    n220 = control-ref of="Elution Countdown (min)"() -> (w297:refnum<vi>)
                    n221 = control-ref of="Current Temp:"() -> (w295:refnum<vi>)
                    n222 = control-ref of="Sparge Countdown (min)"() -> (w299:refnum<vi>)
                    n223 = control-ref of="Sparging Progress Bar"() -> (w298:refnum<vi>)
                    n224 = control-ref of="Current Analyte:"() -> (w292:refnum<vi>)
                    n225 = call "DMS_main_VI_BM.vi"("Constants"=w294, "Metadata"=w293, "Skip sample handling"=FALSE, "Sparging Countdown Timer Refnum"=w299, "Sample Params"=w303, "Sparging Progress Bar Refnum"=w298, "Pump Parameters"=w302, "Mode Selection"=w291, "Elution Countdown Timer Refnum"=w297, "Analysis Type"=w301, "Current Analyte Refnum"=w292, "Temp Refnum"=w295, "Elution Progress Bar Refnum"=w296) -> ()  [unwired: 3 in]
                  }
                  frame "DMS/O" {
                    n226 = local read "Pump Parameters"() -> (w305:T8)
                    n227 = local read "Mode Selection"() -> (w304:T1)
                    n228 = local read "Sample Params"() -> (w316:T6)
                    n229 = local read "Analysis Type"() -> (w317:T3)
                    n230 = local read "Metadata"() -> (w307:T5)
                    n231 = local read "Constants"() -> (w308:T7)
                    n232 = control-ref of="Sparge Countdown (min)"() -> (w313:refnum<vi>)
                    n233 = control-ref of="Reduction Countdown (min)"() -> (w315:refnum<vi>)
                    n234 = control-ref of="Elution Progress Bar"() -> (w311:refnum<vi>)
                    n235 = control-ref of="Elution Countdown (min)"() -> (w310:refnum<vi>)
                    n236 = control-ref of="Current Temp:"() -> (w309:refnum<vi>)
                    n237 = control-ref of="Reduction Progress Bar"() -> (w314:refnum<vi>)
                    n238 = control-ref of="Sparging Progress Bar"() -> (w312:refnum<vi>)
                    n239 = control-ref of="Current Analyte:"() -> (w306:refnum<vi>)
                    n240 = call "DMSO_EC_main_glass_cell_BM.vi"("Constants"=w308, "Reduction Countdown Timer Refnum"=w315, "Metadata"=w307, "Reduction Progress Bar Refnum"=w314, "Sparging Countdown Timer Refnum"=w313, "Sample Params"=w316, "Sparging Progress Bar Refnum"=w312, "Pump Parameters"=w305, "Mode Selection"=w304, "Elution Countdown Timer Refnum"=w310, "Analysis Type"=w317, "Current Analyte Refnum"=w306, "Temp Refnum"=w309, "Elution Progress Bar Refnum"=w311) -> ()  [unwired: 2 in]
                  }
                  frame "DMS/P" {
                    n241 = local read "Metadata"() -> (w321:T5)
                    n242 = local read "Pump Parameters"() -> (w319:T8)
                    n243 = local read "Mode Selection"() -> (w318:T1)
                    n244 = local read "Sample Params"() -> (w330:T6)
                    n245 = control-ref of="Hydrolysis Countdown (min)"() -> (w326:refnum<vi>)
                    n246 = control-ref of="Sparge Countdown (min)"() -> (w324:refnum<vi>)
                    n247 = control-ref of="Elution Progress Bar"() -> (w328:refnum<vi>)
                    n248 = control-ref of="Elution Countdown (min)"() -> (w329:refnum<vi>)
                    n249 = control-ref of="Current Temp:"() -> (w323:refnum<vi>)
                    n250 = local read "Analysis Type"() -> (w331:T3)
                    n251 = control-ref of="Hydrolysis Progress Bar"() -> (w327:refnum<vi>)
                    n252 = control-ref of="Sparging Progress Bar"() -> (w325:refnum<vi>)
                    n253 = local read "Constants"() -> (w322:T7)
                    n254 = control-ref of="Current Analyte:"() -> (w320:refnum<vi>)
                    n255 = call "DMSP_main_VI_BM.vi"("Constants"=w322, "Hydrolysis Countdown Refnum"=w326, "Metadata"=w321, "Hydrolysis Progress Bar Refnum"=w327, "Sparge Countdown Timer Refnum"=w324, "Sample Params"=w330, "Sparging Progress Bar Refnum"=w325, "Pump Parameters"=w319, "Mode Selection"=w318, "Elution Countdown Timer Refnum"=w329, "Analysis Type"=w331, "Current Analyte Refnum"=w320, "Temp Refnum"=w323, "Elution Progress Bar Refnum"=w328) -> ()  [unwired: 2 in]
                  }
                  frame "DMS/O/P" {
                    # "DMS is run first within the DMSP VI procedure"
                    n256 = control-ref of="Reduction Progress Bar"() -> (w340:refnum<vi>)
                    n257 = control-ref of="Reduction Countdown (min)"() -> (w342:refnum<vi>)
                    n258 = control-ref of="Hydrolysis Progress Bar"() -> (w344:refnum<vi>)
                    n259 = local read "Metadata"() -> (w334:T5)
                    n260 = control-ref of="Hydrolysis Countdown (min)"() -> (w345:refnum<vi>)
                    n261 = local read "Pump Parameters"() -> (w347:T8)
                    n262 = local read "Mode Selection"() -> (w332:T1)
                    n263 = local read "Sample Params"() -> (w348:T6)
                    n264 = local read "Analysis Type"() -> (w346:T3)
                    n265 = local read "Constants"() -> (w349:T7)
                    n266 = control-ref of="Elution Countdown (min)"() -> (w338:refnum<vi>)
                    n267 = control-ref of="Elution Progress Bar"() -> (w339:refnum<vi>)
                    n268 = control-ref of="Sparging Progress Bar"() -> (w337:refnum<vi>)
                    n269 = control-ref of="Current Temp:"() -> (w335:refnum<vi>)
                    n270 = control-ref of="Sparge Countdown (min)"() -> (w336:refnum<vi>)
                    n271 = flat-sequence {
                      tunnel: w349 -> [w354]
                      tunnel: w348 -> [w365]
                      tunnel: w347 -> [w351]
                      tunnel: w346 -> [w364]
                      tunnel: w345 -> [w363]
                      tunnel: w344 -> [w362]
                      tunnel: [w361] -> _
                      tunnel: [w361] -> w343
                      tunnel: w342 -> [w361]
                      tunnel: w340 -> [w360]
                      tunnel: [w360] -> w341
                      tunnel: w336 -> [w359]
                      tunnel: w337 -> [w358]
                      tunnel: w338 -> [w357]
                      tunnel: w339 -> [w356]
                      tunnel: w335 -> [w355]
                      tunnel: w334 -> [w353]
                      tunnel: [w353] -> w333
                      tunnel: w332 -> [w350]
                      tunnel: w349 -> [w370]
                      tunnel: w348 -> [w379]
                      tunnel: w347 -> [w367]
                      tunnel: w346 -> [w378]
                      tunnel: w343 -> [w377]
                      tunnel: w341 -> [w376]
                      tunnel: w339 -> [w375]
                      tunnel: w338 -> [w374]
                      tunnel: w337 -> [w373]
                      tunnel: w336 -> [w372]
                      tunnel: w335 -> [w371]
                      tunnel: w333 -> [w369]
                      tunnel: w332 -> [w366]
                      frame #0 {
                        n272 = control-ref of="Current Analyte:"() -> (w352:refnum<vi>)
                        n273 = call "DMSO_EC_main_glass_cell_BM.vi"("Constants"=w354, "Reduction Countdown Timer Refnum"=w363, "Metadata"=w353, "Reduction Progress Bar Refnum"=w362, "Sparging Countdown Timer Refnum"=w359, "Sample Params"=w365, "Sparging Progress Bar Refnum"=w358, "Pump Parameters"=w351, "Mode Selection"=w350, "Elution Countdown Timer Refnum"=w357, "Analysis Type"=w364, "Current Analyte Refnum"=w352, "Temp Refnum"=w355, "Elution Progress Bar Refnum"=w356) -> ()  [unwired: 2 in]
                      }
                      frame #1 {
                        n274 = control-ref of="Current Analyte:"() -> (w368:refnum<vi>)
                        n275 = call "DMSP_main_VI_BM.vi"("Constants"=w370, "Hydrolysis Countdown Refnum"=w377, "Metadata"=w369, "Hydrolysis Progress Bar Refnum"=w376, "Sparge Countdown Timer Refnum"=w372, "Sample Params"=w379, "Sparging Progress Bar Refnum"=w373, "Pump Parameters"=w367, "Mode Selection"=w366, "Elution Countdown Timer Refnum"=w374, "Analysis Type"=w378, "Current Analyte Refnum"=w368, "Temp Refnum"=w371, "Elution Progress Bar Refnum"=w375) -> ()  [unwired: 2 in]
                      }
                    }
                  }
                  frame "DMSO Only" {
                    n276 = local read "Pump Parameters"() -> (w381:T8)
                    n277 = local read "Sample Params"() -> (w392:T6)
                    n278 = local read "Mode Selection"() -> (w380:T1)
                    n279 = local read "Analysis Type"() -> (w393:T3)
                    n280 = local read "Metadata"() -> (w383:T5)
                    n281 = local read "Constants"() -> (w384:T7)
                    n282 = control-ref of="Elution Countdown (min)"() -> (w386:refnum<vi>)
                    n283 = control-ref of="Sparge Countdown (min)"() -> (w389:refnum<vi>)
                    n284 = control-ref of="Reduction Countdown (min)"() -> (w391:refnum<vi>)
                    n285 = control-ref of="Current Temp:"() -> (w385:refnum<vi>)
                    n286 = control-ref of="Reduction Progress Bar"() -> (w390:refnum<vi>)
                    n287 = control-ref of="Sparging Progress Bar"() -> (w388:refnum<vi>)
                    n288 = control-ref of="Elution Progress Bar"() -> (w387:refnum<vi>)
                    n289 = control-ref of="Current Analyte:"() -> (w382:refnum<vi>)
                    n290 = call "DMSO_EC_main_glass_cell_BM.vi"("Constants"=w384, "Reduction Countdown Timer Refnum"=w391, "Metadata"=w383, "Reduction Progress Bar Refnum"=w390, "Sparging Countdown Timer Refnum"=w389, "Sample Params"=w392, "Sparging Progress Bar Refnum"=w388, "Pump Parameters"=w381, "Mode Selection"=w380, "Elution Countdown Timer Refnum"=w386, "Analysis Type"=w393, "Current Analyte Refnum"=w382, "Temp Refnum"=w385, "Elution Progress Bar Refnum"=w387) -> ()  [unwired: 2 in]
                  }
                }
              }
            }
          }
        }
      }
      frame #2 {
        # "Control plotting trap heating"
        n291 = global write "OSSCAR_stop_global_BM.vi" "OSSCAR_stop"(TRUE ("OSSCAR_stop")) -> ()
      }
    }
    n292 = flat-sequence {
      frame #0 {
        # "Plot the trap heating, using data passed through refnums from subVIs"
        n293 = while {
          stop <- w18 stop-if-true
          # "Plot the trap heating"
          n294 = global read "Plot_trap_heating_global_BM.vi" "Plot trap heating"() -> (w17:bool)
          n295 = case shown="True" w17 {
            frame False {
              # "Do nothing when the trap isn't heating"
            }
            frame True {
              n296 = flat-sequence {
                tunnel: [w23] -> w19
                tunnel: w19 -> [w43]
                frame #0 {
                  # "Set tab control to show heating plot"
                  n297 = local write "Tab Control"(T4."Trap Heating" ("Tab Control 2")) -> ()
                }
                frame #1 {
                  # "Plot the trap heating"
                  n298 = Initialize Array(0.0 ("element")) -> (w21:dbl[])  [unwired: 1 in]
                  n299 = while {
                    shift-right: [w30] -> w23
                    shift-left: w21 -> [w32]
                    shift-right: [w25] -> _
                    shift-left: w21 -> [w27]
                    stop <- w37 stop-if-true
                    n300 = call "Elapsed Time"() -> ("Elapsed Time (s)"=w28:dbl)  [unwired: 12 in, 7 out]
                    n301 = local read "Current Temp:"() -> (w39:i32)
                    n302 = global read "Plot_trap_heating_global_BM.vi" "Plot trap heating"() -> (w36:bool)
                    n303 = To Double Precision Float(number=w39) -> (double precision float=w33:dbl)
                    n304 = Build Array (concatenate)(w27, w28) -> (w25:dbl[])
                    n305 = Build Array (concatenate)(w32, w33) -> (w30:dbl[])
                    n306 = Equal?(x=w36, y=FALSE) -> (x = y?=w34:bool)
                    n307 = call "Convert to Dynamic Data2"("Array"=w25) -> ("Dynamic Data Type"=w26:dynamicdata)  [unwired: 3 in]
                    n308 = call "Convert to Dynamic Data"("Array"=w30) -> ("Dynamic Data Type"=w29:dynamicdata)  [unwired: 3 in]
                    n309 = global read "OSSCAR_stop_global_BM.vi" "OSSCAR_stop"() -> (w38:bool)
                    n310 = call "Build XY Graph"("Y Input"=w29, "X Input"=w26) -> ("XY Graph"=→"Trap Heating":cluster{"X":dbl[], "Y":dbl[]}[])  [unwired: 8 in, 1 out]
                    n311 = Or(x=w38, y=w34) -> (x .or. y?=w37:bool)
                    n312 = Wait (ms)(milliseconds to wait=u32 100) -> ()  [unwired: 1 out]
                  }
                }
                frame #2 {
                  # "Record the initial, max, and final temps"
                  n313 = local read "Metadata"() -> (w48:T5)
                  n314 = Array Size(array=w43) -> (size(s)=w45:i32)
                  n315 = Index Array(array=w43, index=0) -> (element=w42:dbl)
                  n316 = Array Max & Min(array=w43) -> (max value=w41:dbl)  [unwired: 3 out]
                  n317 = Decrement(x=w45) -> (x-1=w44:i32)
                  n318 = Index Array(array=w43, index=w44) -> (element=w40:dbl)
                  n319 = global write "Temp_global_BM.vi" "Max Temp (oC)"(w41) -> ()
                  n320 = global write "Temp_global_BM.vi" "Final Temp (oC)"(w40) -> ()
                  n321 = global write "Temp_global_BM.vi" "Intial Temp (oC)"(w42) -> ()
                  n322 = Bundle By Name(cluster=w48, "Initial Trap Temp (oC)"=w42, "Max Trap Temp (oC)"=w41, "Final Trap Temp (oC)"=w40) -> (w46:T5)
                  n323 = local write "Metadata"(w46) -> ()
                }
              }
            }
          }
          n324 = global read "OSSCAR_stop_global_BM.vi" "OSSCAR_stop"() -> (w18:bool)
        }
      }
      frame #1 {
        # "Set tab control to show main outputs"
        n325 = local write "Tab Control"(T4."Metadata" ("Tab Control 2")) -> ()
      }
    }
    n326 = local read "Runtype"() -> (w16:enum16{"Single", "Continuous"})
    n327 = case shown="\"Single\", Default" w16 {
      tunnel: w15 -> [w51 _]
      tunnel: [w50 FALSE] -> w13
      frame "Single", Default {
        # "Stop after 1 iteration"
        n328 = Equal?(x=w51, y=0.0) -> (x = y?=w50:bool)
      }
      frame "Continuous" {
        # "Program is stopped manually by user"
      }
    }
    n329 = global read "Global_stop.vi" "Global Stop"() -> (w12:bool)
    n330 = Or(x=w12, y=w13) -> (x .or. y?=w14:bool)
  }
  n331 = local write "Program Control"(FALSE) -> ()
